vi "test_generic.vi"() -> ()   [LabVIEW 2010, in "GenericSignalWriter.lvclass"]
uses:
  GenericSignalWriter.lvclass
  common/classes/ErrorController/ErrorController/ErrorController.lvclass
  common/classes/ErrorController/ErrorController/class_data.vi
  common/classes/GenericComponent/GenericComponent/GenericComponent.lvclass
panel:
  in  "create button 2":bool
  out "error loaded?":bool
  in  "create button 1":bool
  in  "repetitions":i32=-1 caption="(set to -1 for continuous output)" min=0
  in  "buffer size":i32=360 min=0
  in  "sample dwell time":dbl[unit]=9.999999999999999e-05 caption="(only needed to calculate lag)"
  in  "stop":bool
  in  "start output":bool
  out "Waveform Graph":dbl[](graph)
  # "Test SignalWriter components"
  # "To be specified BEFORE starting this VI:"
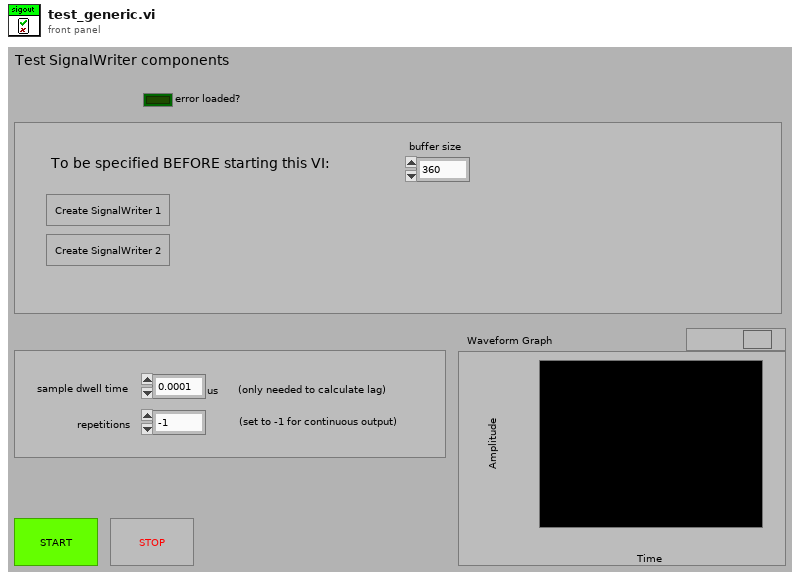
[diagram p1: front panel]
types:
  T1 = typedef "XComponentSpecification.xctl/data.ctl" = cluster{"class path":string, "configuration":string, "label":string, "settings name":string}
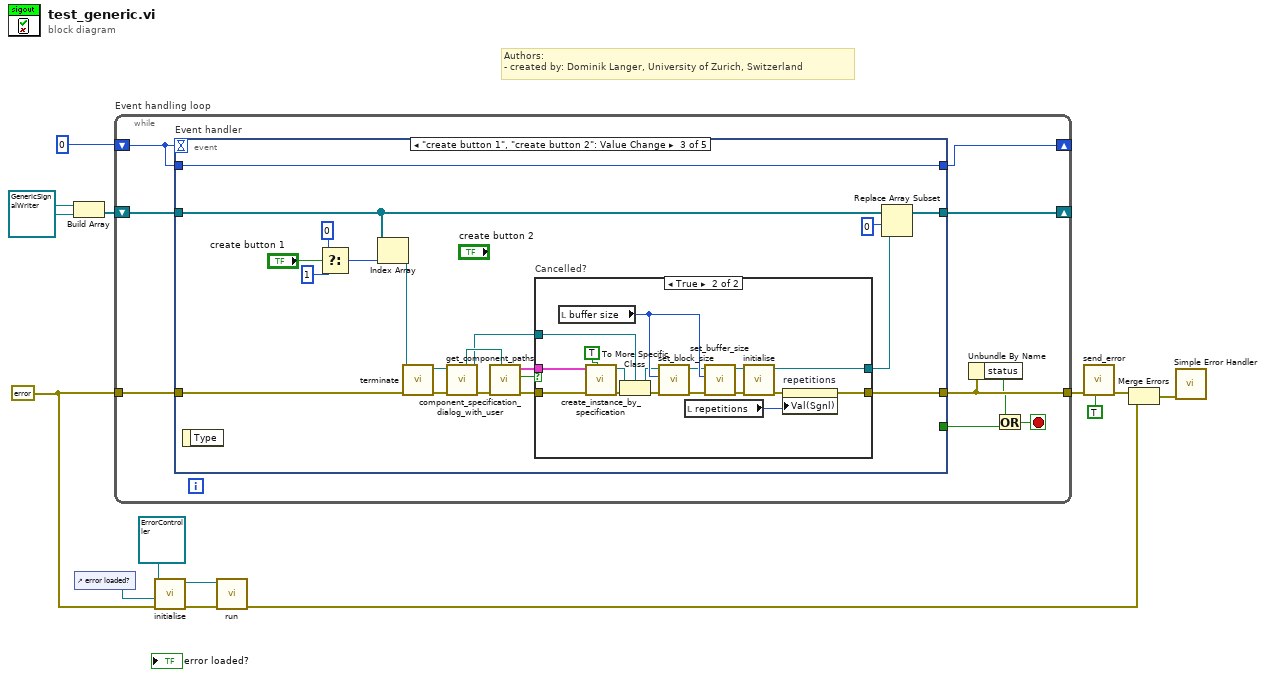
[diagram p0: block diagram]
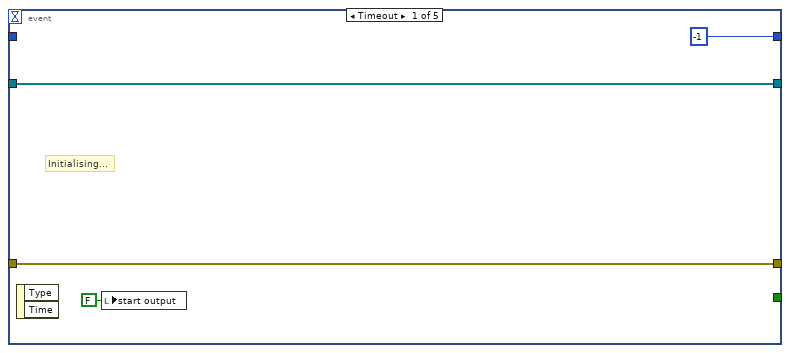
[diagram p2: hidden frame]
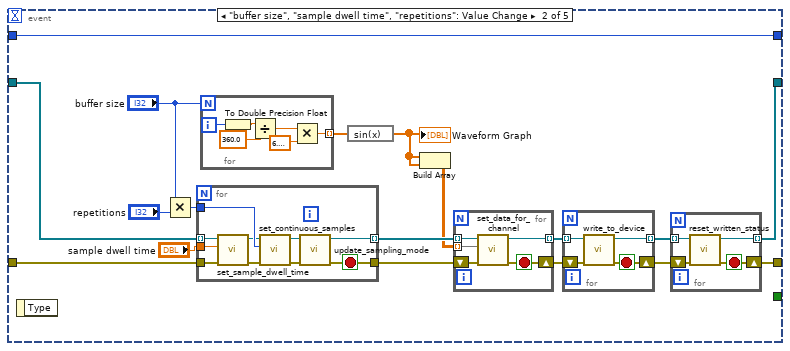
[diagram p3: hidden frame]
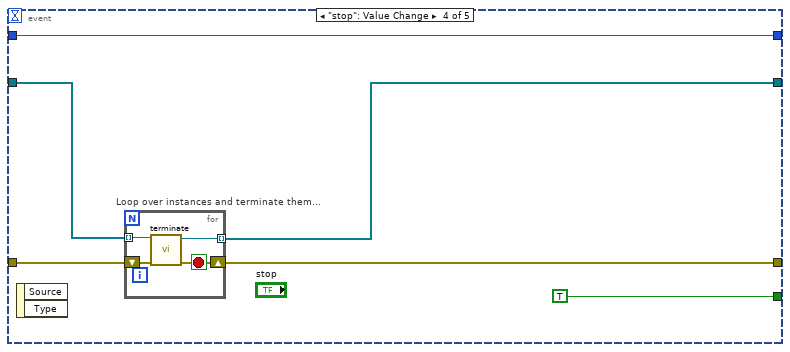
[diagram p5: hidden frame]
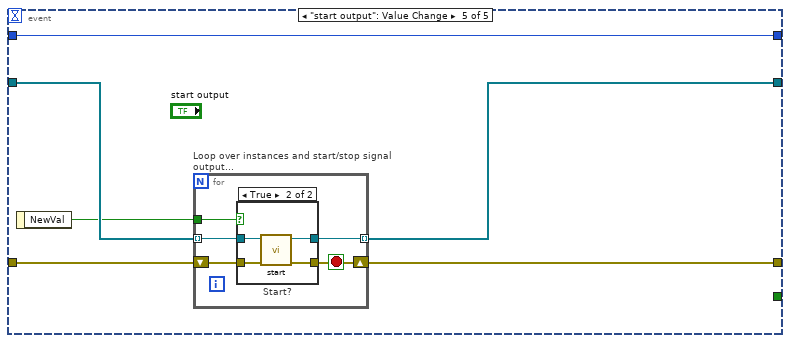
[diagram p6: hidden frame]
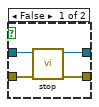
[diagram p7: hidden frame]
diagram:
  w2 = refnum<class "GenericSignalWriter.lvclass"> refnum ("GenericSignalWriter.lvclass")
  w3 = errorcluster {"status"=FALSE, "code"=0, "source"=""} ("error out")
  # "Authors: \n- created by: Dominik Langer, University of Zurich, Switzerland"
  n1 = Build Array(w2, w2) -> (w1:refnum<class "GenericSignalWriter.lvclass">[])
  n2 = control-ref of="error loaded?"() -> (w10:refnum<vi>)
  n3 = while "Event handling loop" {
    shift-right: [w20] -> _
    shift-left: w1 -> [w21]
    shift-right: [w18] -> _
    shift-left: 0 -> [w19]
    tunnel: w3 -> [w22]
    tunnel: [w17] -> w6
    stop <- w14 stop-if-true
    n4 = event "Event handler" shown="[2] \"create button 1\", \"create button 2\": Value Change" {
      selector: _ -> [_ _ _ _ _]
      dyn-events: _ -> [_ _ _ _ _]
      timeout: w19 -> [_ _ _ _ _]
      tunnel: w22 -> [w23 w43 w91 w117 w128]
      tunnel: w21 -> [w24 w42 w84 w115 w127]
      tunnel: [w23 w39 w92 w116 w125] -> w17
      tunnel: [w24 w32 w83 w114 w126] -> w20
      tunnel: [_ _ _ TRUE _] -> w15
      tunnel: [-1 w44 w93 w113 w123] -> w18
      tunnel: w19 -> [_ w44 w93 w113 w123]
      event Timeout {
        # "Initialising..."
        n5 = event-data() -> ()  [unwired: 3 out]
        n6 = local write "start output"(FALSE ("start output")) -> ()
      }
      event "buffer size", "sample dwell time", "repetitions": Value Change {
        n7 = event-data() -> ()  [unwired: 2 out]
        n8 = Multiply(x="buffer size", y="repetitions") -> (x*y=w29:i32)
        n9 = for {
          tunnel: w42 -> [w67] mode=indexing
          tunnel: [w73] -> w35 mode=indexing
          tunnel: "sample dwell time" -> [w68]
          tunnel: w29 -> [w70]
          tunnel: w43 -> [w69]
          tunnel: [w64] -> w37
          stop <- w64 stop-if-true
          n10 = call-dynamic "set_sample_dwell_time.vi"("error in (no error)"=w69, "sample dwell time"=w68, "GenericWriteSignals.lvclass in"=w67) -> ("error out"=w65:errorcluster, "GenericWriteSignals.lvclass out"=w66:refnum<class "GenericSignalWriter.lvclass">)  [unwired: 7 out]
          n11 = call-dynamic "set_continuous_samples.vi"("error in (no error)"=w65, "continuous samples"=w70, "GenericWriteSignals.lvclass in"=w66) -> ("error out"=w72:errorcluster, "GenericWriteSignals.lvclass out"=w71:refnum<class "GenericSignalWriter.lvclass">)  [unwired: 7 out]
          n12 = call-dynamic "update_sampling_mode.vi"("error in (no error)"=w72, "GenericWriteSignals in"=w71) -> ("error out"=w64:errorcluster, "GenericWriteSignals out"=w73:refnum<class "GenericSignalWriter.lvclass">)  [unwired: 8 out]
        }
        n13 = for {
          N: "buffer size" -> [_]
          tunnel: [w45] -> w31 mode=indexing
          i -> [w49]
          n14 = To Double Precision Float(number=w49) -> (double precision float=w50:dbl)
          n15 = Divide(x=w50, y=360.0) -> (x/y=w47:dbl)
          n16 = Multiply(x=w47, y=6.283185307179586) -> (x*y=w45:dbl)
        }
        n17 = expression code="sin(x)"(w31) -> (w30:dbl[])
        "Waveform Graph" <- w30
        n18 = Build Array(w30, w30) -> (w33:dbl[][])
        n19 = for {
          tunnel: w35 -> [w54] mode=indexing
          tunnel: [w53] -> w34 mode=indexing
          tunnel: w33 -> [w52] mode=indexing
          shift-right: [w51] -> w36
          shift-left: w37 -> [w55]
          stop <- w51 stop-if-true
          n20 = call-dynamic "set_data_for_channel.vi"("error in (no error)"=w55, "data"=w52, "GenericWriteSignals in"=w54) -> ("error out"=w51:errorcluster, "GenericWriteSignals out"=w53:refnum<class "GenericSignalWriter.lvclass">)  [unwired: 7 out]
        }
        n21 = for {
          tunnel: [w58] -> w40 mode=indexing
          tunnel: w34 -> [w57] mode=indexing
          shift-right: [w56] -> w41
          shift-left: w36 -> [w59]
          stop <- w56 stop-if-true
          n22 = call-dynamic "write_to_device.vi"("error in (no error)"=w59, "GenericWriteSignals in"=w57) -> ("error out"=w56:errorcluster, "GenericWriteSignals out"=w58:refnum<class "GenericSignalWriter.lvclass">)  [unwired: 1 in, 7 out]
        }
        n23 = for {
          tunnel: w40 -> [w62] mode=indexing
          tunnel: [w61] -> w32 mode=indexing
          shift-right: [w60] -> w39
          shift-left: w41 -> [w63]
          stop <- w60 stop-if-true
          n24 = call-dynamic "reset_written_status.vi"("error in (no error)"=w63, "GenericWriteSignals in"=w62) -> ("error out"=w60:errorcluster, "GenericWriteSignals out"=w61:refnum<class "GenericSignalWriter.lvclass">)  [unwired: 8 out]
        }
      }
      event "create button 1", "create button 2": Value Change {
        n25 = event-data() -> ()  [unwired: 2 out]
        n26 = Select(t=0, s="create button 1", f=1) -> (s? t:f=w74:i32)
        n27 = Index Array(array=w84, index=w74) -> (element=w90:refnum<class "GenericSignalWriter.lvclass">)
        n28 = call-dynamic "terminate.vi"("error in (no error)"=w91, "GenericPlugin in"=w90) -> ("error out"=w87:errorcluster, "GenericPlugin out"=w89:refnum<class "GenericSignalWriter.lvclass">)  [unwired: 8 in]
        n29 = call-dynamic "get_component_paths.vi"("error in (no error)"=w87, "GenericComponent in"=w89) -> ("error out"=w88:errorcluster, "GenericComponent out"=w80:refnum<class "GenericSignalWriter.lvclass">, "component type directory"=w85:path)  [unwired: 4 in, 3 out]
        n30 = call "component_specification_dialog_with_user.vi"("start path"=w85, "error in (no error)"=w88) -> ("error out"=w86:errorcluster, "cancelled?"=w79:bool, "component specification out"=w78:T1)  [unwired: 7 in]
        n31 = case "Cancelled?" shown="True" w79 {
          tunnel: [w95 w112] -> w81
          tunnel: [w94 w109] -> w92
          tunnel: w86 -> [w94 w97]
          tunnel: w80 -> [w95 w96]
          tunnel: w78 -> [_ w98]
          frame False {
          }
          frame True {
            n32 = local read "buffer size"() -> (w108:i32)
            n33 = call "create_instance_by_specification.vi"("call constructor?"=TRUE, "error in (no error)"=w97, "component specification"=w98) -> ("error out"=w101:errorcluster, "GenericPlugin out"=w99:refnum<class "GenericComponent.lvclass">)  [unwired: 6 in, 1 out]
            n34 = To More Specific Class(target class=w96, reference=w99, error in=w101) -> (specific class reference=w100:refnum<class "GenericSignalWriter.lvclass">, error out=w102:errorcluster)
            n35 = call "set_block_size.vi"("error in (no error)"=w102, "block size (samples)"=w108, "GenericWriteSignals.lvclass in"=w100) -> ("error out"=w104:errorcluster, "GenericWriteSignals.lvclass out"=w107:refnum<class "GenericSignalWriter.lvclass">)  [unwired: 7 out]
            n36 = local read "repetitions"() -> (w111:i32)
            n37 = call-dynamic "set_buffer_size.vi"("error in (no error)"=w104, "buffer size (samples)"=w108, "GenericWriteSignals.lvclass in"=w107) -> ("error out"=w105:errorcluster, "GenericWriteSignals.lvclass out"=w106:refnum<class "GenericSignalWriter.lvclass">)  [unwired: 7 out]
            n38 = call-dynamic "initialise.vi"("error in (no error)"=w105, "GenericPlugin in"=w106) -> ("error out"=w110:errorcluster, "GenericPlugin out"=w112:refnum<class "GenericSignalWriter.lvclass">)  [unwired: 8 out]
            n39 = property on="repetitions" class="DigNum (strict)"(error in=w110, "Val(Sgnl)"=w111) -> (error out=w109:errorcluster)  [unwired: 1 in, 1 out]
          }
        }
        n40 = Replace Array Subset(array=w84, new element=w81, index=0) -> (w83:refnum<class "GenericSignalWriter.lvclass">[])
      }
      event "stop": Value Change {
        n41 = event-data() -> ()  [unwired: 3 out]
        n42 = for "Loop over instances and terminate them..." {
          tunnel: w115 -> [w121] mode=indexing
          tunnel: [w120] -> w114 mode=indexing
          shift-right: [w119] -> w116
          shift-left: w117 -> [w122]
          stop <- w119 stop-if-true
          n43 = call-dynamic "terminate.vi"("error in (no error)"=w122, "GenericPlugin in"=w121) -> ("error out"=w119:errorcluster, "GenericPlugin out"=w120:refnum<class "GenericSignalWriter.lvclass">)  [unwired: 8 out]
        }
      }
      event "start output": Value Change {
        n44 = event-data() -> ("NewVal"=w124:bool)  [unwired: 1 out]
        n45 = for "Loop over instances and start/stop signal output..." {
          tunnel: w127 -> [w132] mode=indexing
          shift-right: [w129] -> w125
          shift-left: w128 -> [w133]
          tunnel: [w131] -> w126 mode=indexing
          tunnel: w124 -> [w130]
          stop <- w129 stop-if-true
          n46 = case "Start?" shown="True" w130 {
            tunnel: w133 -> [w137 w141]
            tunnel: w132 -> [w136 w140]
            tunnel: [w134 w139] -> w129
            tunnel: [w135 w138] -> w131
            frame False {
              n47 = call-dynamic "stop.vi"("error in (no error)"=w137, "WriteSignalsGenericPlugin in"=w136) -> ("error out"=w134:errorcluster, "WriteSignalsGenericPlugin out"=w135:refnum<class "GenericSignalWriter.lvclass">)  [unwired: 8 out]
            }
            frame True {
              n48 = call-dynamic "start.vi"("error in (no error)"=w141, "WriteSignalsGenericPlugin in"=w140) -> ("error out"=w139:errorcluster, "WriteSignalsGenericPlugin out"=w138:refnum<class "GenericSignalWriter.lvclass">)  [unwired: 8 out]
            }
          }
        }
      }
    }
    n49 = Unbundle By Name(w17) -> ("status"=w16:bool)
    n50 = Or(x=w16, y=w15) -> (x .or. y?=w14:bool)
  }
  n51 = call-dynamic "initialise.vi"("error in (no error)"=w3, "error boolean"=w10, "ErrorController in"=refnum<class "ErrorController.lvclass"> refnum ("ErrorController.lvclass")) -> ("error out"=w12:errorcluster, "ErrorController out"=w11:refnum<class "ErrorController.lvclass">)  [unwired: 7 in]
  n52 = call "run.vi"("error in (no error)"=w12, "ErrorController in"=w11) -> ("error out"=w8:errorcluster)  [unwired: 8 in, 1 out]
  n53 = call "send_error.vi"("last error? (F)"=TRUE, "error in (no error)"=w6) -> ("error out"=w5:errorcluster)  [unwired: 9 in]
  n54 = Merge Errors(w5, w8) -> (w7:errorcluster)
  n55 = call <vilib>:"Simple Error Handler.vi"("error in (no error)"=w7) -> ()  [unwired: 4 in, 5 out]
